vi "Measurement Logic.vi"(8 "error in":errorcluster, 9 "measurement configuration":T2={"Automation Test"=FALSE, "Power sequencing file path"="", "SMU name"="", "SMU channel"="0", "Compression_Expected DUT Gain (dB)"=17.5, "Compression_Max Linear Range (dBm)"=-10.0, "Compression_Compression Point (dB)"=1.0, "Compression_Target Pin (dBm)"=1.0, "Compression_RFSG Frequency Start (Hz)"=10000000000.0, "Compression_RFSG Frequency Stop (Hz)"=18000000000.0, "Compression_RFSG Number of Frequency Step"=10, "Compression_RFSG Power Start (dBm)"=-20.0, "Compression_RFSG Power Stop(dBm)"=1.0, "Compression_RFSG Power Step Size (dB)"=4.0, "Compression_RBW (Hz)"=0.0} {"Compression_Target Pin (dBm)" format="%#pdBm"}, 10 "measure call context in":refnum<class "Measure Call Context.lvclass">) -> (0 "error out":errorcluster, 1 "measurement results":T1, 2 "measure call context out":refnum<class "Measure Call Context.lvclass">)   [LabVIEW 2023, in "FPT Framework.lvclass"]
doc: "Contains the core logic for executing the measurement."
uses:
  FPT Framework.lvclass
  <vilib>/Plug-In SDKs/Measurements/Measure Call Context/Measure Call Context.lvclass
  Measurement Configuration.ctl
  Measurement Results.ctl
  <vilib>/Analysis/baseanly.llb/Mean (DBL).vi
  <extravilib>/ChannelInstances/Event Messenger-bool/Instantiate.vi
  <vilib>/Analysis/NI_AALBase.lvlib
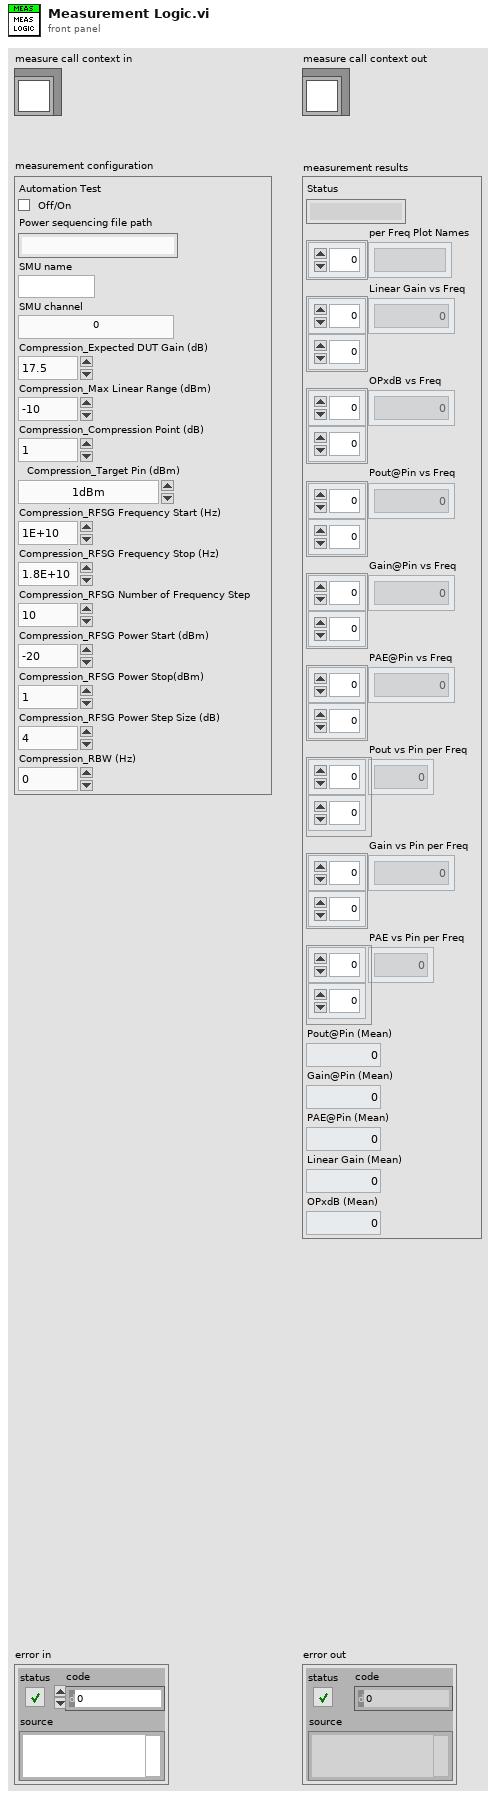
[diagram p1: front panel]
types:
  T1 = typedef "FPT Framework.lvclass/Measurement Results.ctl" = cluster{"Status":string, "per Freq Plot Names":string[], "Linear Gain vs Freq":dbl[][], "OPxdB vs Freq":dbl[][], "Pout@Pin vs Freq":dbl[][], "Gain@Pin vs Freq":dbl[][], "PAE@Pin vs Freq":dbl[][], "Pout vs Pin per Freq":dbl[][], "Gain vs Pin per Freq":dbl[][], "PAE vs Pin per Freq":dbl[][], "Pout@Pin (Mean)":dbl, "Gain@Pin (Mean)":dbl, "PAE@Pin (Mean)":dbl, "Linear Gain (Mean)":dbl, "OPxdB (Mean)":dbl}
  T2 = typedef "FPT Framework.lvclass/Measurement Configuration.ctl" = cluster{"Automation Test":bool, "Power sequencing file path":string, "SMU name":string, "SMU channel":string, "Compression_Expected DUT Gain (dB)":dbl, "Compression_Max Linear Range (dBm)":dbl, "Compression_Compression Point (dB)":dbl, "Compression_Target Pin (dBm)":dbl, "Compression_RFSG Frequency Start (Hz)":dbl, "Compression_RFSG Frequency Stop (Hz)":dbl, "Compression_RFSG Number of Frequency Step":i32, "Compression_RFSG Power Start (dBm)":dbl, "Compression_RFSG Power Stop(dBm)":dbl, "Compression_RFSG Power Step Size (dB)":dbl, "Compression_RBW (Hz)":dbl}
  T3 = enum32{"Power On Dut", "De-embedding + Measurement", "Power Off Dut"}[]
  T4 = cluster{"measurement configuration":T2, "measurement results":T1}
  T5 = typedef "Test Config - Compression.ctl" = cluster{"Expected DUT Gain (dB)":dbl, "Max Linear Range (dBm)":dbl, "Compression Point (dB)":dbl, "Pout at Pin (dBm)":dbl, "RFSG Frequency Start (Hz)":dbl, "RFSG Frequency Stop (Hz)":dbl, "RFSG Number of Frequency Step":i32, "Power Start (dBm)":dbl, "Power Stop(dBm)":dbl, "Power Step Size (dB)":dbl, "RBW (Hz)":dbl}
  T6 = typedef "SMU Config - Compression.ctl" = cluster{"SMU Name":refnum<k15>, "SMU Channel":string}
  T7 = typedef "Results - Compression.ctl" = cluster{"Linear Gain vs Freq":dbl[][], "OPxdb vs Freq":dbl[][], "Pout@Pin vs Freq":dbl[][], "Gain@Pin vs Freq":dbl[][], "PAE@Pin vs Freq":dbl[][], "Pout vs Pin per Freq":dbl[][], "Gain vs Pin per Freq":dbl[][], "PAE vs Pin per Freq":dbl[][]}
  T8 = typedef "Event Messenger-bool.lvlib/))Channel.ctl" = refnum<queue>
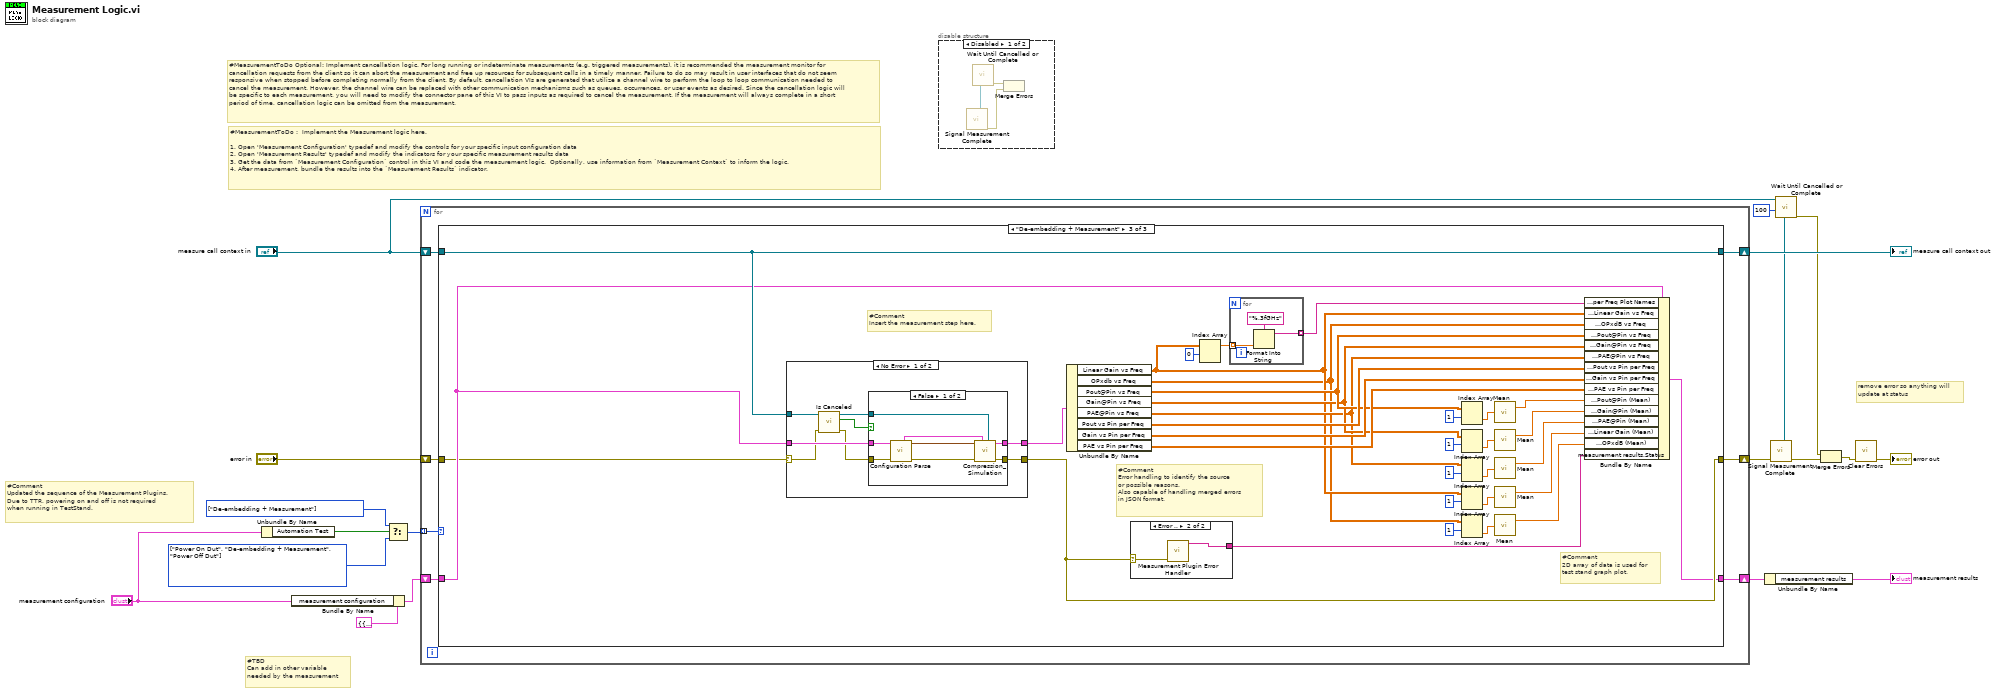
[diagram p0: block diagram]
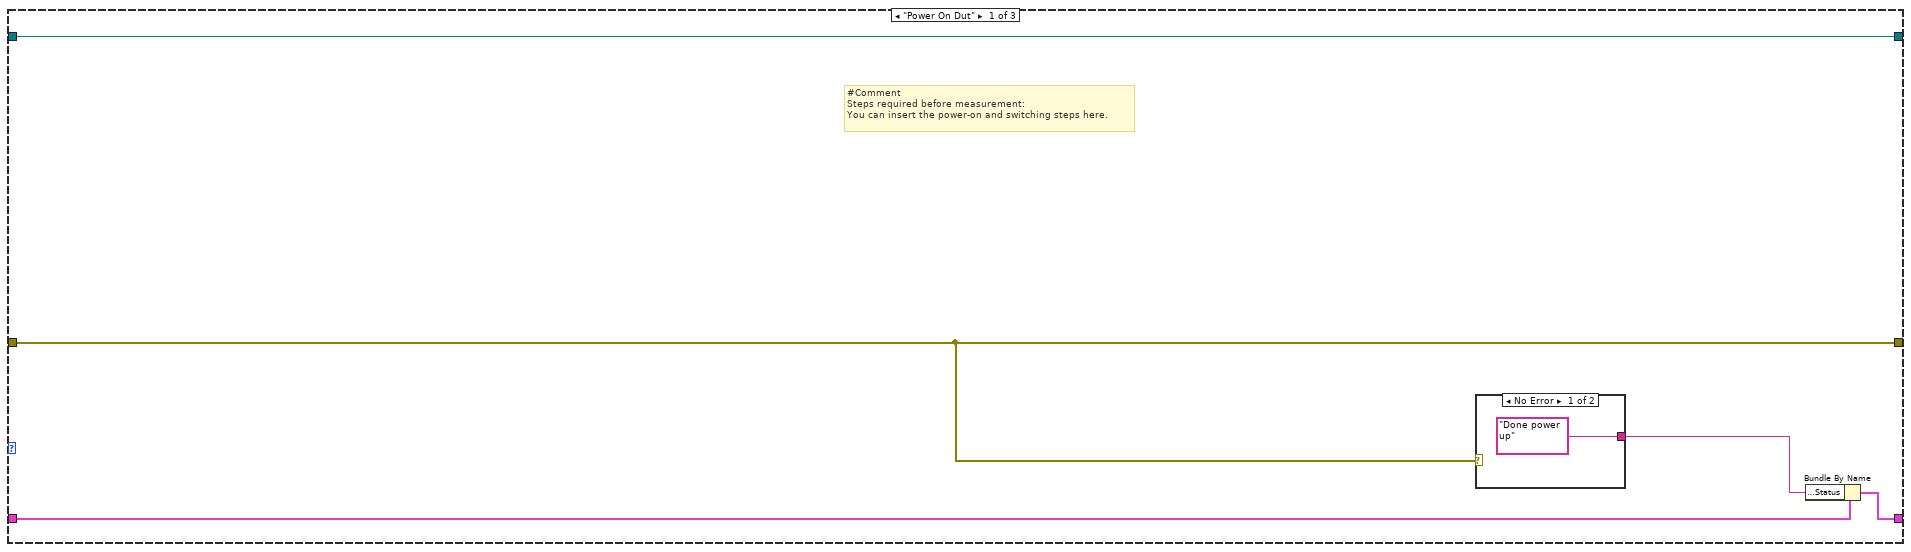
[diagram p2: hidden frame]
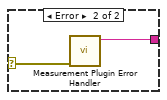
[diagram p3: hidden frame]
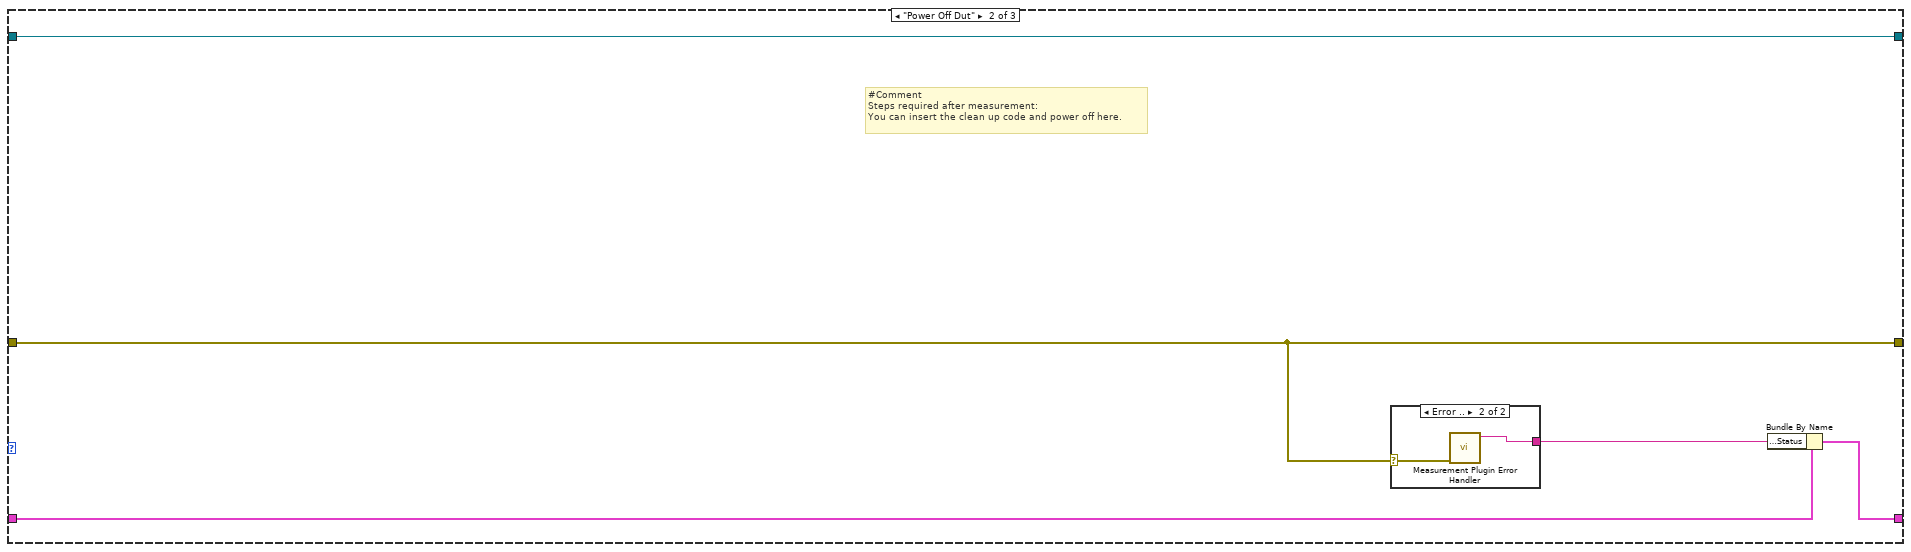
[diagram p4: hidden frame]
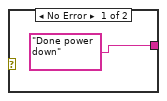
[diagram p5: hidden frame]
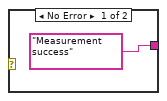
[diagram p6: hidden frame]
diagram:
  w10 = T3 [enum."De-embedding + Measurement"] items=["Power On Dut", "De-embedding + Measurement", "Power Off Dut"]
  w12 = T3 [enum."Power On Dut", enum."De-embedding + Measurement", enum."Power Off Dut"] items=["Power On Dut", "De-embedding + Measurement", "Power Off Dut"]
  # "#Comment\nUpdated the sequence of the Measurement Plugins.\nDue to TTR, powering on and off is not required \nwhen running in TestStand."
  # "remove error so anything will\nupdate at status"
  # "#TBD\nCan add in other variable\nneeded by the measurement"
  # "#MeasurementToDo Optional: Implement cancellation logic. For long running or indeterminate measurements (e.g. triggered measurements), it is recommended the measurement monitor for cancellation requests from the client so it can abort the measurement and free up resources for subsequent calls in a timely manner. Failure to do so may result in user interfaces that do not seem responsive when stopped before completing normally from the client. By default, cancellation VIs are generated that utilize a channel wire to perform the loop to loop communication needed to cancel the measurement. However, the channel wire can be replaced with other communication mechanisms such as queues, occurrences, or user events as desired. Since the cancellation logic will be specific to each measurement, you will need to modify the connector pane of this VI to pass inputs as required to cancel the measurement. If the measurement will always complete in a short period of time, cancellation logic can be omitted from the measurement."
  # "#MeasurementToDo :  Implement the Measurement logic here.\n\n1. Open 'Measurement Configuration' typedef and modify the controls for your specific input configuration data\n2. Open 'Measurement Results' typedef and modify the indicators for your specific measurement results data\n3. Get the data from `Measurement Configuration` control in this VI and code the measurement logic.  Optionally, use information from `Measurement Context` to inform the logic.\n4. After measurement, bundle the results into the `Measurement Results` indicator."
  n1 = Unbundle By Name("measurement configuration") -> ("Automation Test"=w8:bool)
  n2 = Bundle By Name(cluster=T4 {"measurement configuration"={"Automation Test"=FALSE, "Power sequencing file path"="", "SMU name"="", "SMU channel"="0", "Compression_Expected DUT Gain (dB)"=17.5, "Compression_Max Linear Range (dBm)"=-10.0, "Compression_Compression Point (dB)"=1.0, "Compression_Target Pin (dBm)"=1.0, "Compression_RFSG Frequency Start (Hz)"=10000000000.0, "Compression_RFSG Frequency Stop (Hz)"=18000000000.0, "Compression_RFSG Number of Frequency Step"=10, "Compression_RFSG Power Start (dBm)"=-20.0, "Compression_RFSG Power Stop(dBm)"=1.0, "Compression_RFSG Power Step Size (dB)"=4.0, "Compression_RBW (Hz)"=0.0}, "measurement results"={"Status"="", "per Freq Plot Names"=[], "Linear Gain vs Freq"=[], "OPxdB vs Freq"=[], "Pout@Pin vs Freq"=[], "Gain@Pin vs Freq"=[], "PAE@Pin vs Freq"=[], "Pout vs Pin per Freq"=[], "Gain vs Pin per Freq"=[], "PAE vs Pin per Freq"=[], "Pout@Pin (Mean)"=0.0, "Gain@Pin (Mean)"=0.0, "PAE@Pin (Mean)"=0.0, "Linear Gain (Mean)"=0.0, "OPxdB (Mean)"=0.0}}, "measurement configuration"="measurement configuration") -> (w17:T4)
  n3 = Select(t=w10, s=w8, f=w12) -> (s? t:f=w11:T3)
  n4 = for {
    tunnel: w11 -> [w25] mode=indexing
    shift-right: [w20] -> w7
    shift-left: "error in" -> [w26]
    shift-right: [w21] -> w15
    shift-left: w17 -> [w24]
    shift-right: [w22] -> w16
    shift-left: "measure call context in" -> [w23]
    n5 = case shown="\"De-embedding + Measurement\"" w25 {
      tunnel: w26 -> [w31 w35 w43]
      tunnel: w24 -> [w29 w36 w44]
      tunnel: w23 -> [w30 w39 w73]
      tunnel: [w31 w35 w75] -> w20
      tunnel: [w30 w39 w73] -> w22
      tunnel: [w27 w37 w74] -> w21
      frame "Power On Dut" {
        # "#Comment\nSteps required before measurement:\nYou can insert the power-on and switching steps here."
        n6 = case shown="No Error" w31 {
          selector: w31 -> [_ w34]
          tunnel: ["Done power up" w33] -> w28
          frame No Error {
          }
          frame Error {
            n7 = call "Measurement Plugin Error Handler.vi"("error in"=w34) -> ("Status Message (Error)"=w33:string)  [unwired: 9 in, 1 out]
          }
        }
        n8 = Bundle By Name(cluster=w29, "measurement results.Status"=w28) -> (w27:T4)
      }
      frame "Power Off Dut" {
        # "#Comment\nSteps required after measurement:\nYou can insert the clean up code and power off here."
        n9 = case shown="Error .." w35 {
          selector: w35 -> [_ w42]
          tunnel: ["Done power down" w41] -> w38
          frame No Error {
          }
          frame Error {
            n10 = call "Measurement Plugin Error Handler.vi"("error in"=w42) -> ("Status Message (Error)"=w41:string)  [unwired: 9 in, 1 out]
          }
        }
        n11 = Bundle By Name(cluster=w36, "measurement results.Status"=w38) -> (w37:T4)
      }
      frame "De-embedding + Measurement" {
        # "#Comment\nError handling to identify the source \nor possible reasons. \nAlso capable of handling merged errors \nin JSON format."
        # "#Comment\n2D array of data is used for \ntest stand graph plot."
        # "#Comment\nInsert the measurement step here."
        n12 = case shown="No Error" w43 {
          selector: w43 -> [w79 w96]
          tunnel: [w86 w96] -> w75
          tunnel: w73 -> [w85 _]
          tunnel: [w84 _] -> w65
          tunnel: w44 -> [w83 _]
          frame No Error {
            n13 = call <vilib>:"Is Canceled.vi"("error in"=w79, "measure call context in"=w85) -> ("error out"=w80:errorcluster, "is canceled?"=w81:bool, "measure call context out"=w82:refnum<class "Measure Call Context.lvclass">)  [unwired: 7 in]
            n14 = case shown="False" w81 {
              tunnel: [w94 w95] -> w86
              tunnel: w82 -> [w93 _]
              tunnel: [w92 _] -> w84
              tunnel: w83 -> [w91 _]
              tunnel: w80 -> [w90 w95]
              frame False {
                n15 = call "Configuration Parse.vi"("error in"=w90, "UI Controls"=w91) -> ("error out"=w88:errorcluster, "Test Configuration"=w89:T5, "SMU Settings"=w87:T6)  [unwired: 7 in]
                n16 = call "Compression_Simulation.vi"("measure call context in"=w93, "SMU Settings"=w87, "error in"=w88, "Test Configuration"=w89) -> ("error out"=w94:errorcluster, "Data"=w92:T7)  [unwired: 6 in]
              }
              frame True {
              }
            }
          }
          frame Error {
          }
        }
        n17 = Unbundle By Name(w65) -> ("Linear Gain vs Freq"=w51:dbl[][], "OPxdb vs Freq"=w48:dbl[][], "Pout@Pin vs Freq"=w57:dbl[][], "Gain@Pin vs Freq"=w56:dbl[][], "PAE@Pin vs Freq"=w55:dbl[][], "Pout vs Pin per Freq"=w64:dbl[][], "Gain vs Pin per Freq"=w63:dbl[][], "PAE vs Pin per Freq"=w62:dbl[][])
        n18 = case shown="Error .." w75 {
          selector: w75 -> [_ w78]
          tunnel: ["Measurement success" w77] -> w45
          frame No Error {
          }
          frame Error {
            n19 = call "Measurement Plugin Error Handler.vi"("error in"=w78) -> ("Status Message (Error)"=w77:string)  [unwired: 9 in, 1 out]
          }
        }
        n20 = Index Array(array=w51, index (row)=0) -> (element=w69:dbl[])  [unwired: 1 in]
        n21 = for {
          tunnel: w69 -> [w97] mode=indexing
          tunnel: [w98] -> w67 mode=indexing
          # "Get Plot Names"
          n22 = Format Into String(format string="%.3fGHz", w97) -> (resulting string=w98:string)  [unwired: 2 in, 1 out]
        }
        n23 = Index Array(array=w57, index (row)=1) -> (element=w61:dbl[])  [unwired: 1 in]
        n24 = Index Array(array=w56, index (row)=1) -> (element=w58:dbl[])  [unwired: 1 in]
        n25 = Index Array(array=w55, index (row)=1) -> (element=w60:dbl[])  [unwired: 1 in]
        n26 = Index Array(array=w51, index (row)=1) -> (element=w59:dbl[])  [unwired: 1 in]
        n27 = Index Array(array=w48, index (row)=1) -> (element=w50:dbl[])  [unwired: 1 in]
        n28 = call-poly <vilib>:"Mean.vi"("X"=w61) -> ("mean"=w54:dbl)  [unwired: 1 out]
        n29 = call-poly <vilib>:"Mean.vi"("X"=w58) -> ("mean"=w53:dbl)  [unwired: 1 out]
        n30 = call-poly <vilib>:"Mean.vi"("X"=w60) -> ("mean"=w52:dbl)  [unwired: 1 out]
        n31 = call-poly <vilib>:"Mean.vi"("X"=w59) -> ("mean"=w47:dbl)  [unwired: 1 out]
        n32 = call-poly <vilib>:"Mean.vi"("X"=w50) -> ("mean"=w46:dbl)  [unwired: 1 out]
        n33 = Bundle By Name(cluster=w44, "measurement results.per Freq Plot Names"=w67, "measurement results.Linear Gain vs Freq"=w51, "measurement results.OPxdB vs Freq"=w48, "measurement results.Pout@Pin vs Freq"=w57, "measurement results.Gain@Pin vs Freq"=w56, "measurement results.PAE@Pin vs Freq"=w55, "measurement results.Pout vs Pin per Freq"=w64, "measurement results.Gain vs Pin per Freq"=w63, "measurement results.PAE vs Pin per Freq"=w62, "measurement results.Pout@Pin (Mean)"=w54, "measurement results.Gain@Pin (Mean)"=w53, "measurement results.PAE@Pin (Mean)"=w52, "measurement results.Linear Gain (Mean)"=w47, "measurement results.OPxdB (Mean)"=w46, "measurement results.Status"=w45) -> (w74:T4)
      }
    }
  }
  "measure call context out" <- w16
  n34 = disable-structure shown="Disabled" {
    frame Disabled {
      n35 = call "Signal Measurement Complete.vi"() -> ("error out"=w101:errorcluster, "done channel"=w102:T8)  [unwired: 10 in]
      n36 = call "Wait Until Cancelled or Complete.vi"("done channel"=w102) -> ("error out"=w100:errorcluster)  [unwired: 9 in, 1 out]
      n37 = Merge Errors(w100, w101) -> ()  [unwired: 1 out]
    }
    frame Enabled {
    }
  }
  n38 = Unbundle By Name(w15) -> ("measurement results"=→"measurement results":T1)
  n39 = call "Signal Measurement Complete.vi"("error in (no error)"=w7) -> ("error out"=w6:errorcluster, "done channel"=w5:T8)  [unwired: 9 in]
  n40 = call "Wait Until Cancelled or Complete.vi"("done channel"=w5, "ms polling interval"=100, "measure call context in"="measure call context in") -> ("error out"=w1:errorcluster)  [unwired: 7 in, 1 out]
  n41 = Merge Errors(w1, w6) -> (w2:errorcluster)
  n42 = call <vilib>:"Clear Errors.vi"("error in (no error)"=w2) -> ("error out"=→"error out":errorcluster)  [unwired: 5 in, 1 out]
